vi "Get Device Names.vi"(7 "Use Cached Data?":bool, 8 "Error In":errorcluster, 10 "Structure Name":string, 11 "Nest Config":T1) -> (0 "Error Out":errorcluster, 2 "Device Names":string[](array[string]), 3 "Nest Config":T1)   [LabVIEW 2013, in "LVH-Nest.lvlib"]
doc: "Get the names of all of the Nest devices in the specified structure."
uses:
  LVH-Nest.lvlib
  Private/Type Defs/Nest Config.ctl
  <vilib>/httpClient/ClientHandle.ctl
  Private/Type Defs/Session Data.ctl
  <vilib>/httpClient/LabVIEWHTTPClient.lvlib
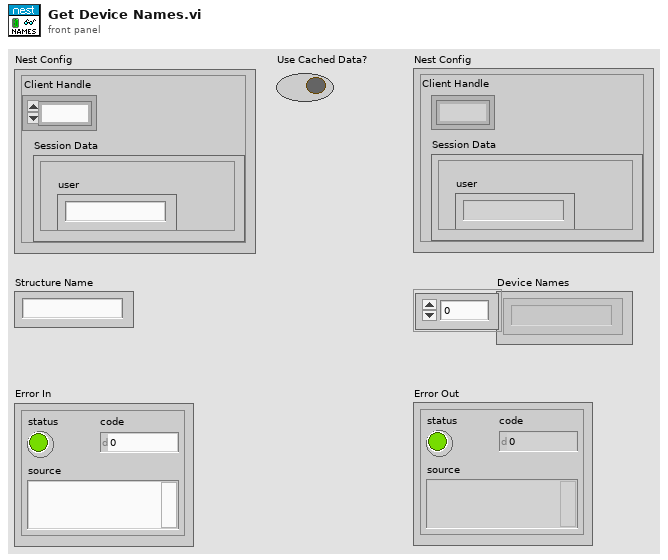
[diagram p1: front panel]
types:
  T1 = typedef "LVH-Nest.lvlib/Nest Config.ctl" = cluster{"Client Handle":T2, "Session Data":T3}
  T2 = typedef "LabVIEWHTTPClient.lvlib/ClientHandle.ctl" = refnum<k1>
  T3 = typedef "LVH-Nest.lvlib/Session Data.ctl" = cluster{"is_superuser":bool, "is_staff":bool, "urls":cluster{"transport_url":string, "rubyapi_url":string, "weather_url":string, "log_upload_url":string, "support_url":string}, "limits":cluster{"thermostats_per_structure":u32, "structures":u32, "thermostats":u32, "smoke_detectors":u32, "smoke_detectors_per_structure":u32}, "access_token":string, "userid":string, "expires_in":string, "email":string, "user":string, "language":string}
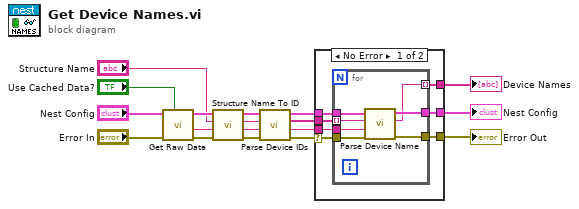
[diagram p0: block diagram]
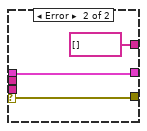
[diagram p2: hidden frame]
diagram:
  n1 = call "Get Raw Data.vi"("Use Cached Data?"="Use Cached Data?", "Error In"="Error In", "Nest Config"="Nest Config") -> ("Error Out"=w16:errorcluster, "Data"=w18:string, "Nest Config"=w17:T1)  [unwired: 6 in]
  n2 = call "Structure Name To ID.vi"("Error In"=w16, "Data"=w18, "Structure Name"="Structure Name", "Nest Config"=w17) -> ("Error Out"=w9:errorcluster, "Data"=w10:string, "Structure ID"=w11:string, "Nest Config"=w8:T1)  [unwired: 4 in]
  n3 = call "Parse Device IDs.vi"("Error In"=w9, "Data"=w10, "Structure ID"=w11, "Nest Config"=w8) -> ("Error Out"=w1:errorcluster, "Data"=w5:string, "Device IDs"=w6:string[], "Nest Config"=w7:T1)  [unwired: 4 in]
  n4 = case shown="No Error" w1 {
    selector: w1 -> [w19 w35]
    tunnel: w7 -> [w25 w34]
    tunnel: w6 -> [w24 _]
    tunnel: w5 -> [w23 _]
    tunnel: [w22 w35] -> w4
    tunnel: [w21 w34] -> w3
    tunnel: [w20 string[] []] -> w2
    frame No Error {
      n5 = for {
        tunnel: w19 -> [w32]
        tunnel: w25 -> [w31]
        tunnel: w24 -> [w30] mode=indexing
        tunnel: w23 -> [w29]
        tunnel: [w27] -> w22
        tunnel: [w28] -> w21
        tunnel: [w26] -> w20 mode=indexing
        n6 = call "Parse Device Name.vi"("Error In"=w32, "Data"=w29, "Device ID"=w30, "Nest Config"=w31) -> ("Error Out"=w27:errorcluster, "Device Name"=w26:string, "Nest Config"=w28:T1)  [unwired: 4 in, 1 out]
      }
    }
    frame Error {
    }
  }
  "Error Out" <- w4
  "Nest Config" <- w3
  "Device Names" <- w2
